vi "ParseSQLiteDescribe.vi"(4 "error in (no error)":errorcluster, 6 "String":string, 7 "Data":string[][](array[string])) -> (0 "error out":errorcluster, 3 "appended array":string[][](array[string]))   [LabVIEW 2023]
doc: "*-----------------------------------------------------\n* Author: SWatts\n*\n* VI Description: Parse dB self description data\n* \n*\n* Error handling: All errors passed out\n*\n* Pre-condition: \n*\n* Post-condition: None\n*\n* Revision History:\n*\n* Rev Date Author Description \n* 01 30/04/2014 SWatts First issue\n*\n*-----------------------------------------------------"
panel:
  # "Input"
  # "Output"
  # "+------------+----------+------+-----+---------+----------------+\n| Field      | Type     | Null | Key | Default | Extra          |\n+------------+----------+------+-----+---------+----------------+\n| Id         | int(11)  | NO   | PRI | NULL    | auto_increment |\n| Name       | char(35) | NO   |     |         |                |\n| Country    | char(3)  | NO   | UNI |         |                |\n| District   | char(20) | YES  | MUL |         |                |\n| Population | int(11)  | NO   |     | 0       |                |\n+------------+----------+------+-----+---------+----------------+"
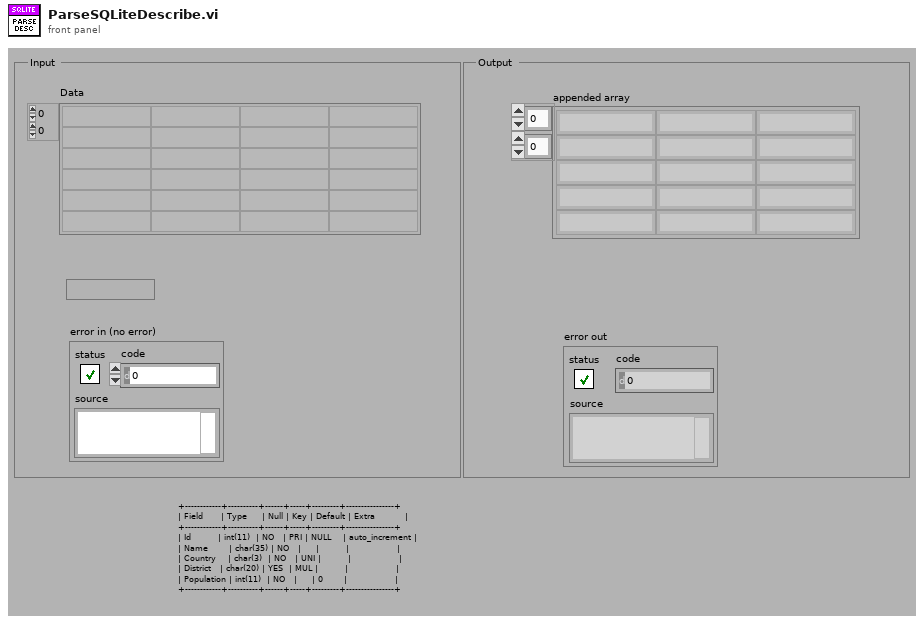
[diagram p1: front panel]
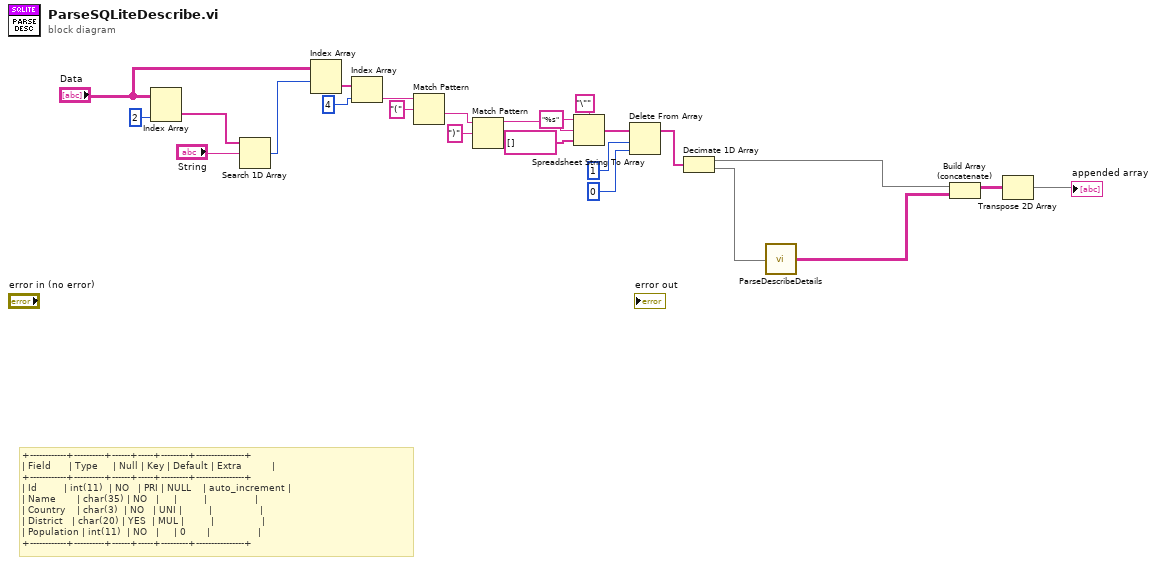
[diagram p0: block diagram]
diagram:
  # "+------------+----------+------+-----+---------+----------------+\n| Field      | Type     | Null | Key | Default | Extra          |\n+------------+----------+------+-----+---------+----------------+\n| Id         | int(11)  | NO   | PRI | NULL    | auto_increment |\n| Name       | char(35) | NO   |     |         |                |\n| Country    | char(3)  | NO   | UNI |         |                |\n| District   | char(20) | YES  | MUL |         |                |\n| Population | int(11)  | NO   |     | 0       |                |\n+------------+----------+------+-----+---------+----------------+"
  n1 = Index Array(array="Data", index (col)=2 ("disabled index (col)")) -> (element=w23:string[])  [unwired: 1 in]
  n2 = Search 1D Array(1D array=w23, element="String") -> (index of element=w20:i32)  [unwired: 1 in]
  n3 = Index Array(array="Data", index (row)=w20) -> (element=w19:string[])  [unwired: 1 in]
  n4 = Index Array(array=w19, index=4) -> (element=w17:string)
  n5 = Match Pattern(string=w17, regular expression="(") -> (after substring=w15:string)  [unwired: 1 in, 3 out]
  n6 = Match Pattern(string=w15, regular expression=")") -> (before substring=w11:string)  [unwired: 1 in, 3 out]
  n7 = Spreadsheet String To Array(delimiter (Tab)="\"", format string="%s", spreadsheet string=w11, array type (2D Dbl)=string[] []) -> (array=w9:string[])
  n8 = Delete From Array(array=w9, length=1, index=0) -> (array with subset deleted=w6:string[])  [unwired: 1 out]
  n9 = Decimate 1D Array(w6) -> (w3:string[], w5:string[])
  n10 = call "ParseDescribeDetails.vi"("DescribeDataIn"=w5) -> ("DescribeData"=w4:string[][])  [unwired: 4 in]
  n11 = Build Array (concatenate)(w3, w4) -> (w2:string[][])
  n12 = Transpose 2D Array(2D array=w2) -> (transposed array=→"appended array":string[][])
